vi "Create plots - ring selector.vi"(6 "Relative time":bool, 7 "Data reduction":T2={"Clip time"=FALSE, "Tiime 0"=0.0, "Time 1"=0.0, "Maximum data points"=1, "Decimation method"=enum."Min-Max"}, 8 "Error In":errorcluster, 10 "File-group-channel":T1(array[cluster]), 11 "Plots  selector":cluster{"X":u16, "Y":u16}[](array[cluster]) {"Y" items=["Select channel...", "Time", "Y"]; "X" items=["Select channel...", "Time", "Y"]}) -> (0 "Error Out":errorcluster, 2 "Plots":cluster{dbl[], dbl[]}[](array[cluster]) {"?" format="%#_10g"})   [LabVIEW 2015]
uses:
  Controls/Data reduction.ctl
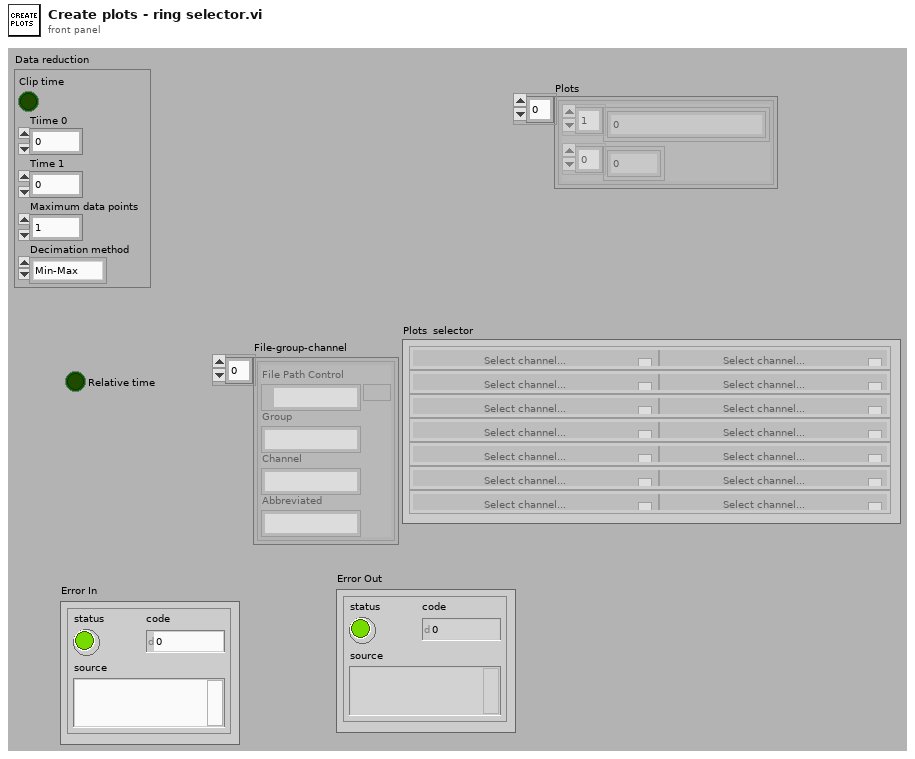
[diagram p1: front panel]
types:
  T1 = cluster{"File Path Control":path, "Group":string, "Channel":string, "Abbreviated":string}[]
  T2 = typedef "Data reduction.ctl" = cluster{"Clip time":bool, "Tiime 0":dbl, "Time 1":dbl, "Maximum data points":i32, "Decimation method":enum16{"coerce", "linear", "spline", "Min-Max", "Average"}}
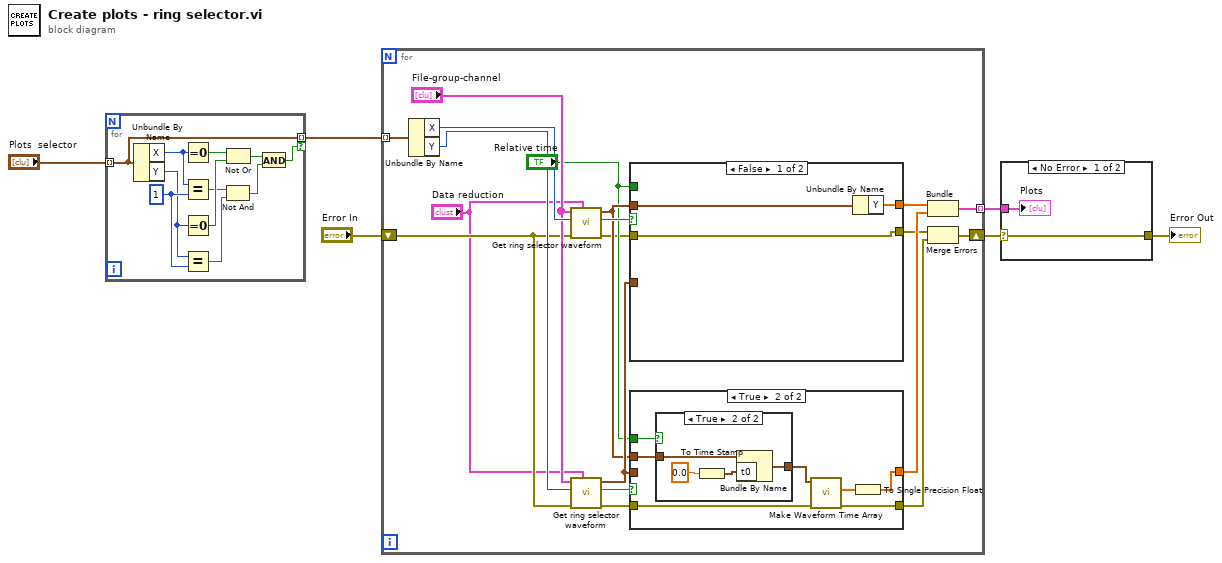
[diagram p0: block diagram]
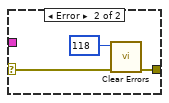
[diagram p2: hidden frame]
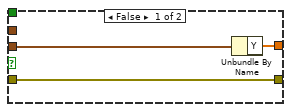
[diagram p3: hidden frame]
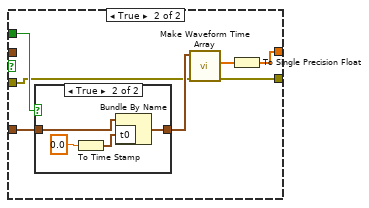
[diagram p5: hidden frame]
diagram:
  n1 = for {
    tunnel: "Plots  selector" -> [w15] mode=indexing
    tunnel: [w15] -> w5 mode=indexing if=w8
    w12 = u16 1 ("y")
    n2 = Unbundle By Name(w15) -> ("X"=w13:u16, "Y"=w11:u16)
    n3 = Equal To 0?(x=w13) -> (x = 0?=w17:bool)
    n4 = Equal?(x=w13, y=w12) -> (x = y?=w10:bool)
    n5 = Equal To 0?(x=w11) -> (x = 0?=w16:bool)
    n6 = Equal?(x=w11, y=w12) -> (x = y?=w9:bool)
    n7 = Not Or(1:w16, 2:w17) -> (0:w14:bool)
    n8 = Not And(1:w9, 2:w10) -> (0:w7:bool)
    n9 = And(x=w14, y=w7) -> (x .and. y?=w8:bool)
  }
  n10 = for {
    tunnel: w5 -> [w36] mode=indexing
    shift-right: [w22] -> w2
    shift-left: "Error In" -> [w21]
    tunnel: [w20] -> w3 mode=indexing
    n11 = Unbundle By Name(w36) -> ("X"=w35:u16, "Y"=w34:u16)
    n12 = call "Get ring selector waveform.vi"("Clip/desimate"="Data reduction", "Error In"=w21, "Channel"=w35, "File-group-channel"="File-group-channel") -> ("Error Out"=w27:errorcluster, "Empty waveform"=w32:bool, "Waveform"=w29:waveform(sgl))  [unwired: 5 in]
    n13 = call "Get ring selector waveform.vi"("Clip/desimate"="Data reduction", "Error In"=w21, "Channel"=w34, "File-group-channel"="File-group-channel") -> ("Error Out"=w26:errorcluster, "Empty waveform"=w18:bool, "Waveform"=w30:waveform(sgl))  [unwired: 5 in]
    n14 = case shown="False" w32 {
      tunnel: w29 -> [w54 _]
      tunnel: [w53 w55] -> w31
      tunnel: w30 -> [_ w60]
      tunnel: "Relative time" -> [_ w61]
      tunnel: [w52 w57] -> w24
      tunnel: w27 -> [w52 w56]
      frame False {
        n15 = Unbundle By Name(w54) -> ("Y"=w53:sgl[])
      }
      frame True {
        n16 = case shown="True" w61 {
          tunnel: w60 -> [w62 w66]
          tunnel: [w62 w65] -> w59
          frame False {
          }
          frame True {
            n17 = To Time Stamp(1:0.0) -> (0:w63:timestamp)
            n18 = Bundle By Name(cluster=w66, "t0"=w63) -> (w65:waveform(sgl))
          }
        }
        n19 = call "Make Waveform Time Array.vi"("error in (no error)"=w56, "waveform in"=w59) -> ("error out"=w57:errorcluster, "X array"=w58:dbl[])  [unwired: 8 in]
        n20 = To Single Precision Float(number=w58) -> (single precision float=w55:sgl[])
      }
    }
    n21 = case shown="True" w18 {
      tunnel: w30 -> [w39 _]
      tunnel: [w38 w40] -> w25
      tunnel: w29 -> [_ w45]
      tunnel: "Relative time" -> [_ w46]
      tunnel: [w37 w42] -> w23
      tunnel: w26 -> [w37 w41]
      frame False {
        n22 = Unbundle By Name(w39) -> ("Y"=w38:sgl[])
      }
      frame True {
        n23 = case shown="True" w46 {
          tunnel: w45 -> [w47 w51]
          tunnel: [w47 w50] -> w44
          frame False {
          }
          frame True {
            n24 = To Time Stamp(1:0.0) -> (0:w48:timestamp)
            n25 = Bundle By Name(cluster=w51, "t0"=w48) -> (w50:waveform(sgl))
          }
        }
        n26 = call "Make Waveform Time Array.vi"("error in (no error)"=w41, "waveform in"=w44) -> ("error out"=w42:errorcluster, "X array"=w43:dbl[])  [unwired: 8 in]
        n27 = To Single Precision Float(number=w43) -> (single precision float=w40:sgl[])
      }
    }
    n28 = Bundle("Y"=w31, "Y"=w25) -> (w20:cluster{"Y":sgl[], "Y":sgl[]})  [unwired: 1 out]
    n29 = Merge Errors(w24, w23) -> (w22:errorcluster)
  }
  n30 = case shown="No Error" w2 {
    selector: w2 -> [w67 w70]
    tunnel: w3 -> [w68 _]
    tunnel: [w67 w69] -> w1
    frame No Error {
      "Plots" <- w68
    }
    frame Error {
      n31 = call <vilib>:"Clear Errors.vi"("error in (no error)"=w70, "specific error code to clear (0: all)"=118) -> ("error out"=w69:errorcluster)  [unwired: 4 in, 1 out]
    }
  }
  "Error Out" <- w1
